vi "State_Machine.vi"(8 "error in (no error)":errorcluster caption="entrée d'erreur (pas d'erreur)", 11 "Delay en entrée":refnum<class "Generate_Install_Code.lvclass">) -> (0 "error out":errorcluster caption="sortie d'erreur", 2 "Json_String":string, 3 "Delay en sortie":refnum<class "Generate_Install_Code.lvclass">)   [LabVIEW 2020, in "Library Test.lvlib" / "Generate_Install_Code.lvclass"]
uses:
  Generate_Install_Code.lvclass
  C:/Users/ngarcin/OneDrive - Altyor/Standard TB/Class/Test/Test (Default)/Test (Default).lvclass
  JSON API/JSON Value/Set from JSON string.vi
  JSON API/JSON Value/JSON Value.lvclass
  Generate_Install_Code.lvclass/Generate_Install_Code.ctl
  JSON API/Variant JSON/Variant JSON.lvlib
  JSON API/Get Polymorphic/JSON GetSet.lvlib
  Commun VI/Library Commun.lvlib
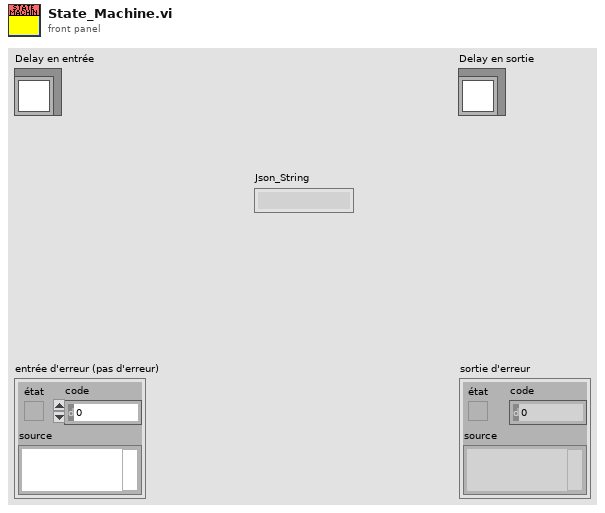
[diagram p1: front panel]
types:
  T1 = enum16{"open", "replace", "create", "open or create", "replace or create", "replace or create with confirmation"}
  T2 = cluster{"Path File InstallCode":path, "Store With CRC":bool}
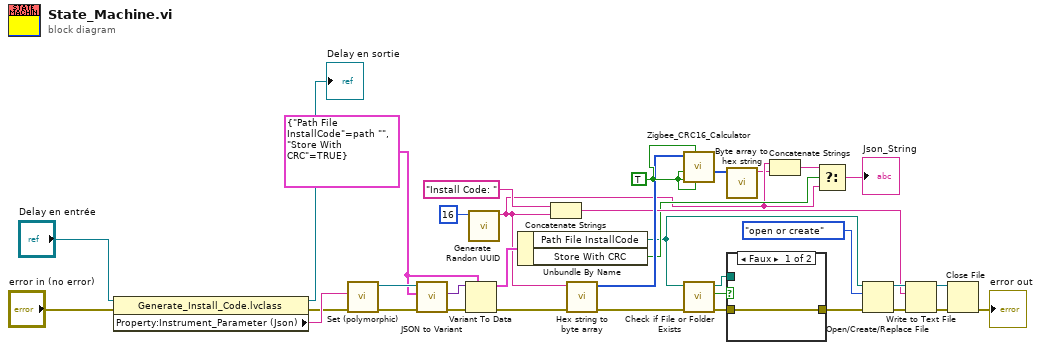
[diagram p0: block diagram]
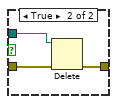
[diagram p2: hidden frame]
diagram:
  w24 = TRUE
  w26 = T2 {"Path File InstallCode"=path "", "Store With CRC"=TRUE}
  n1 = property class="Generate_Install_Code.lvclass"(reference="Delay en entrée", error in="error in (no error)") -> (reference out=→"Delay en sortie":refnum<class "Generate_Install_Code.lvclass">, error out=w27:errorcluster, "Property:Instrument_Parameter (Json)"=w30:string)
  n2 = call-poly "Set (polymorphic).vi"("error in (no error)"=w27, "JSON stream"=w30) -> ("error out"=w32:errorcluster, "JSON Value out"=w34:refnum<class "JSON Value.lvclass">)  [unwired: 7 in, 1 out]
  n3 = call "JSON to Variant.vi"("error in (no error)"=w32, "Variant (Data Type)"=w26, "JSON Value"=w34) -> ("error out"=w33:errorcluster, "Variant out"=w31:variant)  [unwired: 7 in]
  n4 = Variant To Data(error in=w33, type=w26, Variant=w31) -> (data=w8:T2, error out=w21:errorcluster)
  n5 = call "Generate Randon UUID.vi"("Taille"=16) -> ("chaîne"=w3:string)  [unwired: 10 in]
  n6 = Unbundle By Name(w8) -> ("Path File InstallCode"=w6:path, "Store With CRC"=w7:bool)
  n7 = Concatenate Strings("Install Code: " ("chaîne"), w3) -> (w10:string)
  n8 = call "Hex string to byte array.vi"("Error In"=w21, "Hex string"=w3) -> ("Error Out"=w4:errorcluster, "Byte Array"=w22:u8[])  [unwired: 8 in]
  n9 = call "Zigbee_CRC16_Calculator.vi"("ReverseCRC"=w24, "LSB First"=w24, "Postcond"=w24, "Precond"=w24, "Input"=w22) -> ("Bytes"=w23:u8[])  [unwired: 4 in, 2 out]
  n10 = call <vilib>:"Check if File or Folder Exists.vi"("error in (no error)"=w4, "path"=w6) -> ("error out"=w17:errorcluster, "file or folder exists?"=w18:bool, "dup path"=w19:path)  [unwired: 7 in]
  n11 = call "Byte array to hex string.vi"("Array"=w23) -> ("String"=w2:string)  [unwired: 10 in]
  n12 = case shown="Faux" w18 {
    tunnel: w17 -> [w36 w39]
    tunnel: w19 -> [_ w38]
    tunnel: [w36 w37] -> w20
    frame False {
    }
    frame True {
      n13 = Delete(path (use dialog)=w38, error in=w39) -> (error out=w37:errorcluster)  [unwired: 3 in, 2 out]
    }
  }
  n14 = Concatenate Strings(w3, w2) -> (w1:string)
  n15 = Select(t=w1, s=w7, f=w3) -> (s? t:f=→"Json_String":string)
  n16 = Open/Create/Replace File(file path (use dialog)=w6, error in=w20, operation (0:open)=T1."open or create" ("opération (0 : open)")) -> (refnum out=w13:refnum<file>, error out=w14:errorcluster)  [unwired: 3 in, 1 out]
  n17 = Write to Text File(file (use dialog)=w13, text=w10, error in=w14) -> (refnum out=w16:refnum<file>, error out=w15:errorcluster)  [unwired: 1 in, 1 out]
  n18 = Close File(refnum=w16, error in=w15) -> (error out=→"error out":errorcluster)  [unwired: 1 out]
